vi "Do.vi"(8 "error in (no error)":errorcluster, 10 "Actor in":refnum<class "Actor.lvclass">, 11 "Save or Load Config Msg in":refnum<class "Save or Load Config Msg.lvclass">) -> (0 "error out":errorcluster, 2 "Actor out":refnum<class "Actor.lvclass">)   [LabVIEW 2020, in "GUI.lvlib" / "Save or Load Config Msg.lvclass"]
doc: "(<B>Filename</B>: Actor Framework.lvlib:Message.lvclass:Do.vi)\n\nDefines what a message does when it is received by an actor. Generally, a message instructs an actor to invoke one of its methods. By default, this method does nothing. A child class must override it to define behavior. Create a child class by using the Actor Framework Message Maker dialog box."
uses:
  Save or Load Config Msg.lvclass
  <vilib>/ActorFramework/Actor/Actor.lvclass
  GUI/GUI.lvclass
  C:/Program Files/National Instruments/LabVIEW 2020/vi.lib/ActorFramework/Actor/Actor.lvclass
  Save or Load Config Msg.lvclass/Save or Load Config Msg.ctl
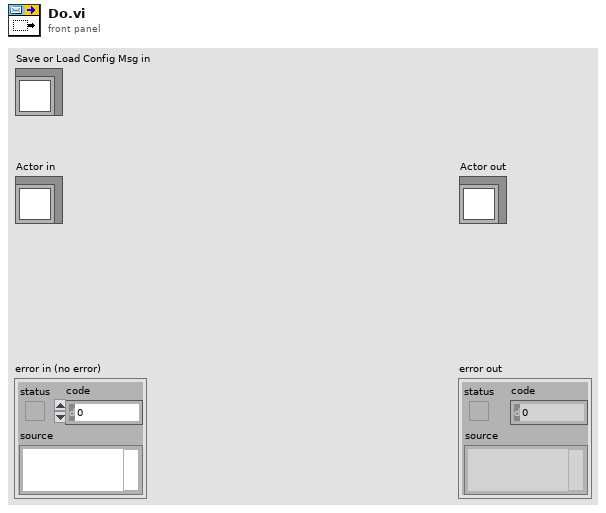
[diagram p1: front panel]
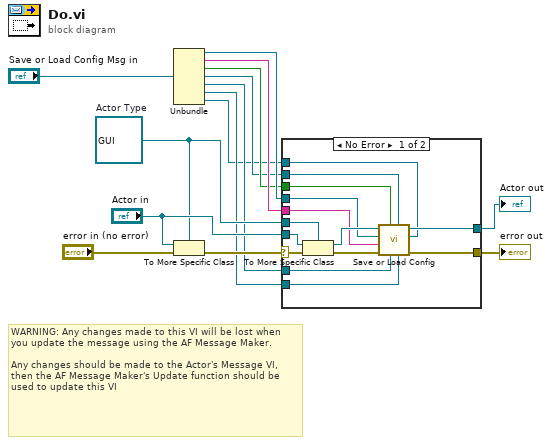
[diagram p0: block diagram]
diagram:
  w9 = refnum<class "GUI.lvclass"> refnum  # Actor Type
  # "WARNING: Any changes made to this VI will be lost when you update the message using the AF Message Maker.\n\nAny changes should be made to the Actor's Message VI, then the AF Message Maker's Update function should be used to update this VI"
  n1 = Unbundle("Save or Load Config Msg in") -> (w8:refnum<vi>, w7:string, w6:bool, w5:refnum<vi>, w4:refnum<vi>, w3:refnum<vi>, w2:refnum<queue>)
  n2 = To More Specific Class(target class=w9, reference="Actor in", error in="error in (no error)") -> (error out=w13:errorcluster)  [unwired: 1 out]
  n3 = case shown="No Error" w13 {
    selector: w13 -> [w28 w30]
    tunnel: [w23 w30] -> w12
    tunnel: [w22 w29] -> w11
    tunnel: "Actor in" -> [w27 w29]
    tunnel: w9 -> [w26 _]
    tunnel: w8 -> [w21 _]
    tunnel: w7 -> [w20 _]
    tunnel: w6 -> [w19 _]
    tunnel: w5 -> [w18 _]
    tunnel: w4 -> [w17 _]
    tunnel: w3 -> [w16 _]
    tunnel: w2 -> [w15 _]
    frame No Error {
      n4 = To More Specific Class ("Actor Cast")(target class=w26, reference=w27, error in=w28) -> (specific class reference=w25:refnum<class "GUI.lvclass">, error out=w24:errorcluster)
      n5 = call "Save or Load Config.vi"("GUI Helper Q"=w15, "Config Select Ref"=w16, "Auto Clust"=w18, "Task Info in"=w17, "Save?"=w19, "error in (no error)"=w24, "Task Configuration Name"=w20, "Task Selection in"=w21, "GUI in"=w25) -> ("error out"=w23:errorcluster, "GUI out"=w22:refnum<class "GUI.lvclass">)  [unwired: 1 in]
    }
    frame Error {
    }
  }
  "error out" <- w12
  "Actor out" <- w11
